vi "ingest.job_result_rid.vi"(8 "error in":errorcluster, 11 "IngestJob in":refnum<class "IngestJob.lvclass">) -> (0 "error out":errorcluster, 3 "IngestJob out":refnum<class "IngestJob.lvclass">)   [LabVIEW 2020, in "IngestJob.lvclass"]
doc: "Returns the identifier of the dataset or video the ingest job produced, if known."
uses:
  IngestJob.lvclass
  IngestJob.lvclass/IngestJob.ctl
  client.lvlib
panel:
  out "out_needed out":u32
  out "result rid":string
  out "is_present out":bool
  in  "out_needed":u32
  in  "cap":u32
  in  "buf":string
  in  "is_present":bool
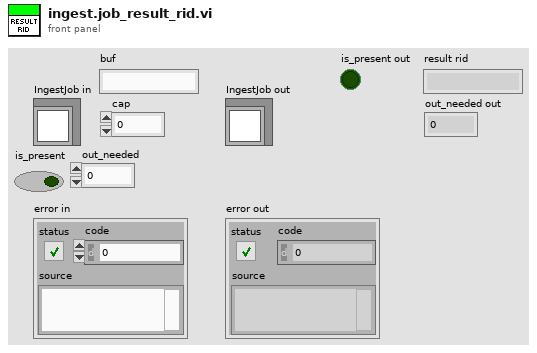
[diagram p1: front panel]
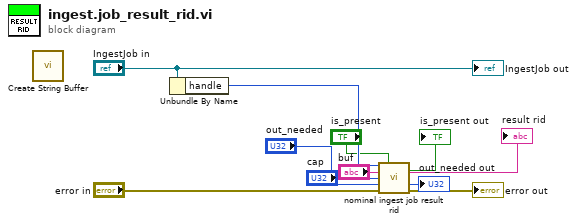
[diagram p0: block diagram]
diagram:
  n1 = call "Create String Buffer.vi"() -> ()  [unwired: 9 in, 3 out]
  n2 = Unbundle By Name("IngestJob in") -> ("handle"=w9:i32)
  n3 = call "nominal ingest job result rid.vi"("job"=w9, "is_present"="is_present", "buf"="buf", "cap"="cap", "out_needed"="out_needed", "error in (no error)"="error in") -> ("is_present out"=→"is_present out":bool, "buf out"=→"result rid":string, "out_needed out"=→"out_needed out":u32, "error out"=→"error out":errorcluster)  [unwired: 5 in, 1 out]
  "IngestJob out" <- "IngestJob in"
